vi "BuildMask_Color.vi"(0 "tolerance":dbl=10.0, 2 "color":u32(colorbox)=16749312, 3 "Image":T1 {"Dialogs" format="%.0b"}) -> (1 "Image":T1 {"Dialogs" format="%.0b"})   [LabVIEW 2010]
doc: "This vi will return a mask. The area inside the defined ROI is filled with 255 and the rest of the image is set to 0."
uses:
  <userlib>/ImageProcessing/QTLIB_2595_LV86/QT_Image.ctl
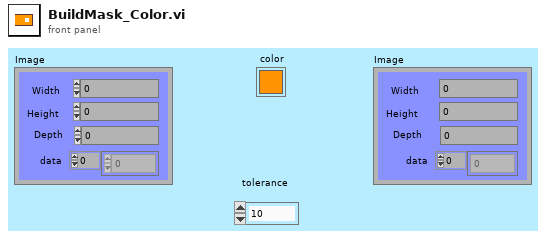
[diagram p1: front panel]
types:
  T1 = typedef "QT_Image.ctl" = cluster{"Width":i32, "Height":i32, "Depth":i32, "data":u8[], "Compressed data":u8[], "Color table":u32[], "Duration":i32, "Options":i32, "Timestamp":i32, "ID":i32, "Reserved":i32, "Dialogs":u32}
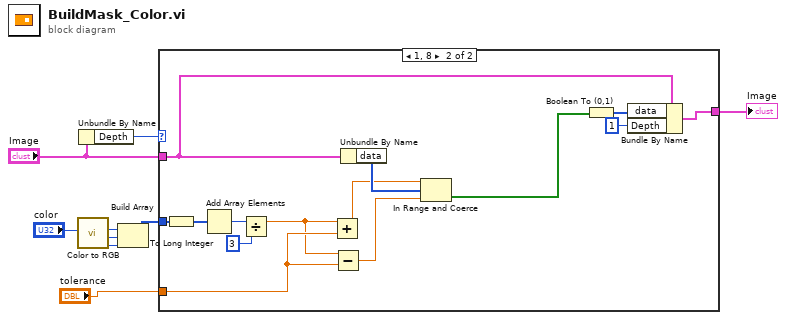
[diagram p0: block diagram]
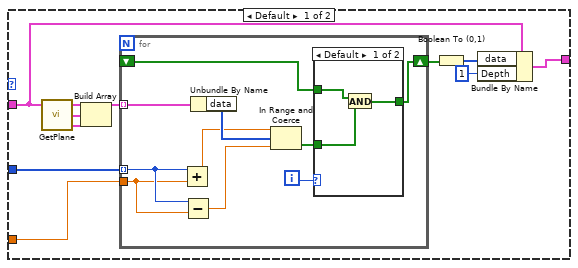
[diagram p2: hidden frame]
diagram:
  n1 = call <vilib>:"Color to RGB.vi"("Color"="color") -> ("R"=w5:u8, "G"=w4:u8, "B"=w3:u8)  [unwired: 1 out]
  n2 = Unbundle By Name("Image") -> ("Depth"=w8:i32)
  n3 = Build Array(w5, w4, w3) -> (w2:u8[])
  n4 = case shown="1, 8" w8 {
    tunnel: [w11 w45] -> w1
    tunnel: "Image" -> [w13 w41]
    tunnel: w2 -> [w20 w48]
    tunnel: "tolerance" -> [w19 w47]
    frame Default {
      n5 = call <userlib>:"GetPlane.vi"("Image In"=w13) -> ("Blue Plane Out"=w16:T1, "Green Plane Out"=w17:T1, "Red Plane Out"=w18:T1)
      n6 = Build Array(w18, w17, w16) -> (w15:T1[])
      n7 = for {
        tunnel: w15 -> [w30] mode=indexing
        tunnel: w20 -> [w28] mode=indexing
        tunnel: w19 -> [w27]
        shift-right: [w23] -> w14
        shift-left: _ -> [w21]
        i -> [w24]
        n8 = Add(x=w28, y=w27) -> (x+y=w26:dbl)
        n9 = Subtract(x=w28, y=w27) -> (x-y=w25:dbl)
        n10 = Unbundle By Name(w30) -> ("data"=w29:u8[])
        n11 = In Range and Coerce(upper limit=w26, x=w29, lower limit=w25) -> (In Range?=w22:bool[])  [unwired: 1 out]
        n12 = case shown="Default" w24 {
          tunnel: [w31 w34] -> w23
          tunnel: w22 -> [w33 w34]
          tunnel: w21 -> [w32 _]
          frame Default {
            n13 = And(x=w32, y=w33) -> (x .and. y?=w31:bool[])
          }
          frame 0 {
          }
        }
      }
      n14 = Boolean To (0,1)(Boolean=w14) -> (0, 1=w12:i16[])
      n15 = Bundle By Name(cluster=w13, "data"=w12, "Depth"=1) -> (w11:T1)
    }
    frame 1, 8 {
      n16 = To Long Integer(number=w48) -> (32bit integer=w36:i32[])
      n17 = Add Array Elements(numeric array=w36) -> (sum=w39:i32)
      n18 = Divide(x=w39, y=3) -> (x/y=w38:dbl)
      n19 = Add(x=w38, y=w47) -> (x+y=w43:dbl)
      n20 = Subtract(x=w38, y=w47) -> (x-y=w42:dbl)
      n21 = Unbundle By Name(w41) -> ("data"=w44:u8[])
      n22 = In Range and Coerce(upper limit=w43, x=w44, lower limit=w42) -> (In Range?=w40:bool[])  [unwired: 1 out]
      n23 = Boolean To (0,1)(Boolean=w40) -> (0, 1=w46:i16[])
      n24 = Bundle By Name(cluster=w41, "data"=w46, "Depth"=1) -> (w45:T1)
    }
  }
  "Image" <- w1
